vi "Get_Deploy_EXE_Data.vi"(8 "error in (no error)":errorcluster, 11 "AB_Deploy_EXE.lvclass in":refnum<class "AB_Deploy_EXE.lvclass">) -> (0 "error out":errorcluster, 2 "data":T1, 3 "AB_Deploy_EXE.lvclass out":refnum<class "AB_Deploy_EXE.lvclass">)   [LabVIEW 2020, in "AB_Deploy_EXE.lvclass"]
uses:
  <vilib>/AppBuilder/AB_Classes/DeployableEXE/AB_Deploy_EXE.lvclass
  <vilib>/AppBuilder/AB_Classes/DeployableEXE/AB_Deploy_EXE.ctl
  <vilib>/AppBuilder/AB_Classes/DeployableEXE/AB_Deploy_EXE.lvclass/AB_Deploy_EXE.ctl
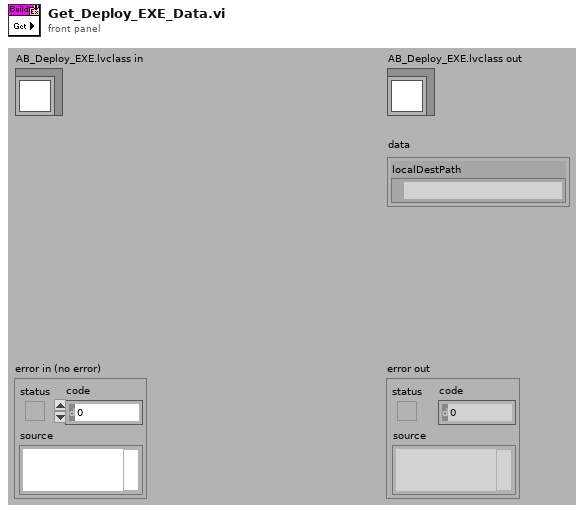
[diagram p1: front panel]
types:
  T1 = typedef "AB_Deploy_EXE.ctl" = cluster{"localDestPath":path}
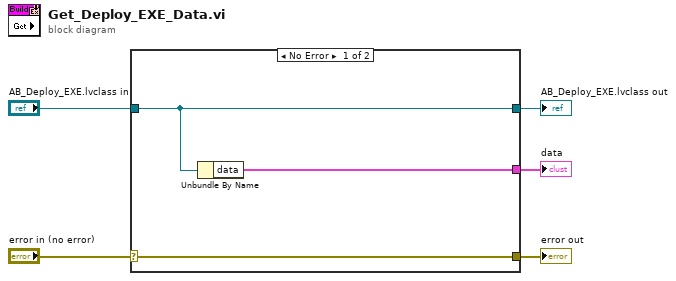
[diagram p0: block diagram]
diagram:
  n1 = case shown="No Error" "error in (no error)" {
    selector: "error in (no error)" -> [w8 w9]
    tunnel: [w8 w9] -> w4
    tunnel: [w7 w10] -> w2
    tunnel: "AB_Deploy_EXE.lvclass in" -> [w7 w10]
    tunnel: [w6 _] -> w1
    frame No Error {
      n2 = Unbundle By Name(w7) -> ("data"=w6:T1)
    }
    frame Error {
    }
  }
  "error out" <- w4
  "AB_Deploy_EXE.lvclass out" <- w2
  "data" <- w1
